vi "language.vi"(8 "Error In":errorcluster, 11 "QLocale In":refnum<class "QLocale.lvclass">) -> (0 "Error Out":errorcluster, 2 "Value":T1 items=["AnyLanguage", "C", "Abkhazian", "Oromo", "Afar", "Afrikaans", "Albanian", "Amharic", "Arabic", "Armenian", "Assamese", "Aymara", "Azerbaijani", "Bashkir", "Basque", "Bengali", "Dzongkha", "Bihari", "Bislama", "Breton", "Bulgarian", "Burmese", "Belarusian", "Khmer", "Catalan", "Chinese", "Corsican", "Croatian", "Czech", "Danish", "Dutch", "English", "Esperanto", "Estonian", "Faroese", "Fijian", "Finnish", "French", "WesternFrisian", "Gaelic", "Galician", "Georgian", "German", "Greek", "Greenlandic", "Guarani", "Gujarati", "Hausa", "Hebrew", "Hindi", "Hungarian", "Icelandic", "Indonesian", "Interlingua", "Interlingue", "Inuktitut", "Inupiak", "Irish", "Italian", "Japanese", "Javanese", "Kannada", "Kashmiri", "Kazakh", "Kinyarwanda", "Kirghiz", "Korean", "Kurdish", "Rundi", "Lao", "Latin", "Latvian", "Lingala", "Lithuanian", "Macedonian", "Malagasy", "Malay", "Malayalam", "Maltese", "Maori", "Marathi", "Marshallese", "Mongolian", "NauruLanguage", "Nepali", "NorwegianBokmal", "Occitan", "Oriya", "Pashto", "Persian", "Polish", "Portuguese", "Punjabi", "Quechua", "Romansh", "Romanian", "Russian", "Samoan", "Sango", "Sanskrit", "Serbian", "Ossetic", "SouthernSotho", "Tswana", "Shona", "Sindhi", "Sinhala", "Swati", "Slovak", "Slovenian", "Somali", "Spanish", "Sundanese", "Swahili", "Swedish", "Sardinian", "Tajik", "Tamil", "Tatar", "Telugu", "Thai", "Tibetan", "Tigrinya", "Tongan", "Tsonga", "Turkish", "Turkmen", "Tahitian", "Uighur", "Ukrainian", "Urdu", "Uzbek", "Vietnamese", "Volapuk", "Welsh", "Wolof", "Xhosa", "Yiddish", "Yoruba", "Zhuang", "Zulu", "NorwegianNynorsk", "Bosnian", "Divehi", "Manx", "Cornish", "Akan", "Konkani", "Ga", "Igbo", "Kamba", "Syriac", "Blin", "Geez", "Koro", "Sidamo", "Atsam", "Tigre", "Jju", "Friulian", "Venda", "Ewe", "Walamo", "Hawaiian", "Tyap", "Nyanja", "Filipino", "SwissGerman", "SichuanYi", "Kpelle", "LowGerman", "SouthNdebele", "NorthernSotho", "NorthernSami", "Taroko", "Gusii", "Taita", "Fulah", "Kikuyu", "Samburu", "Sena", "NorthNdebele", "Rombo", "Tachelhit", "Kabyle", "Nyankole", "Bena", "Vunjo", "Bambara", "Embu", "Cherokee", "Morisyen", "Makonde", "Langi", "Ganda", "Bemba", "Kabuverdianu", "Meru", "Kalenjin", "Nama", "Machame", "Colognian", "Masai", "Soga", "Luyia", "Asu", "Teso", "Saho", "KoyraChiini", "Rwa", "Luo", "Chiga", "CentralMoroccoTamazight", "KoyraboroSenni", "Shambala", "Bodo", "Avaric", "Chamorro", "Chechen", "Church", "Chuvash", "Cree", "Haitian", "Herero", "HiriMotu", "Kanuri", "Komi", "Kongo", "Kwanyama", "Limburgish", "LubaKatanga", "Luxembourgish", "Navaho", "Ndonga", "Ojibwa", "Pali", "Walloon", "Aghem", "Basaa", "Zarma", "Duala", "JolaFonyi", "Ewondo", "Bafia", "MakhuwaMeetto", "Mundang", "Kwasio", "Nuer", "Sakha", "Sangu", "CongoSwahili", "Tasawaq", "Vai", "Walser", "Yangben", "Avestan", "Asturian", "Ngomba", "Kako", "Meta", "Ngiemboon", "Aragonese", "Akkadian", "AncientEgyptian", "AncientGreek", "Aramaic", "Balinese", "Bamun", "BatakToba", "Buginese", "Buhid", "Carian", "Chakma", "ClassicalMandaic", "Coptic", "Dogri", "EasternCham", "EasternKayah", "Etruscan", "Gothic", "Hanunoo", "Ingush", "LargeFloweryMiao", "Lepcha", "Limbu", "Lisu", "Lu", "Lycian", "Lydian", "Mandingo", "Manipuri", "Meroitic", "NorthernThai", "OldIrish", "OldNorse", "OldPersian", "OldTurkish", "Pahlavi", "Parthian", "Phoenician", "PrakritLanguage", "Rejang", "Sabaean", "Samaritan", "Santali", "Saurashtra", "Sora", "Sylheti", "Tagbanwa", "TaiDam", "TaiNua", "Ugaritic", "Akoose", "Lakota", "StandardMoroccanTamazight", "Mapuche", "CentralKurdish", "LowerSorbian", "UpperSorbian", "Kenyang", "Mohawk", "Nko", "Prussian", "Kiche", "SouthernSami", "LuleSami", "InariSami", "SkoltSami", "Warlpiri", "ManichaeanMiddlePersian", "Mende", "AncientNorthArabian", "LinearA", "HmongNjua", "Ho", "Lezghian", "Bassa", "Mono", "TedimChin", "Maithili", "Ahom", "AmericanSignLanguage", "ArdhamagadhiPrakrit", "Bhojpuri", "HieroglyphicLuwian", "LiteraryChinese", "Mazanderani", "Mru", "Newari", "NorthernLuri", "Palauan", "Papiamento", "Saraiki", "TokelauLanguage", "TokPisin", "TuvaluLanguage", "UncodedLanguages", "Cantonese", "Osage", "Tangut"], 3 "QLocale Out":refnum<class "QLocale.lvclass">)   [LabVIEW 2014, in "QLocale.lvclass"]
doc: "LabVIEW-specific documentation is not yet available. See <b>https://doc.qt.io/qt-5/qlocale.html#language</b>"
uses:
  QLocale.lvclass
  Language.ctl
  LQSerialData/LQSerialData.lvclass/LQSerialData.ctl
  LQ Core.lvlib
  LQSerialData/LQSerialData.lvclass
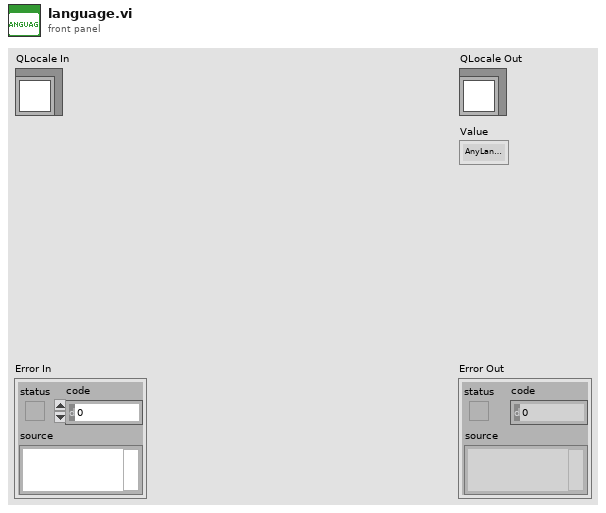
[diagram p1: front panel]
types:
  T1 = typedef "QLocale.lvclass/Language.ctl" = i32
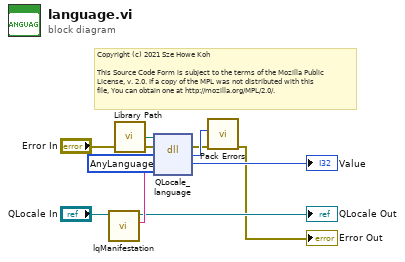
[diagram p0: block diagram]
diagram:
  w8 = T1 0 items=["AnyLanguage", "C", "Abkhazian", "Oromo", "Afar", "Afrikaans", "Albanian", "Amharic", "Arabic", "Armenian", "Assamese", "Aymara", "Azerbaijani", "Bashkir", "Basque", "Bengali", "Dzongkha", "Bihari", "Bislama", "Breton", "Bulgarian", "Burmese", "Belarusian", "Khmer", "Catalan", "Chinese", "Corsican", "Croatian", "Czech", "Danish", "Dutch", "English", "Esperanto", "Estonian", "Faroese", "Fijian", "Finnish", "French", "WesternFrisian", "Gaelic", "Galician", "Georgian", "German", "Greek", "Greenlandic", "Guarani", "Gujarati", "Hausa", "Hebrew", "Hindi", "Hungarian", "Icelandic", "Indonesian", "Interlingua", "Interlingue", "Inuktitut", "Inupiak", "Irish", "Italian", "Japanese", "Javanese", "Kannada", "Kashmiri", "Kazakh", "Kinyarwanda", "Kirghiz", "Korean", "Kurdish", "Rundi", "Lao", "Latin", "Latvian", "Lingala", "Lithuanian", "Macedonian", "Malagasy", "Malay", "Malayalam", "Maltese", "Maori", "Marathi", "Marshallese", "Mongolian", "NauruLanguage", "Nepali", "NorwegianBokmal", "Occitan", "Oriya", "Pashto", "Persian", "Polish", "Portuguese", "Punjabi", "Quechua", "Romansh", "Romanian", "Russian", "Samoan", "Sango", "Sanskrit", "Serbian", "Ossetic", "SouthernSotho", "Tswana", "Shona", "Sindhi", "Sinhala", "Swati", "Slovak", "Slovenian", "Somali", "Spanish", "Sundanese", "Swahili", "Swedish", "Sardinian", "Tajik", "Tamil", "Tatar", "Telugu", "Thai", "Tibetan", "Tigrinya", "Tongan", "Tsonga", "Turkish", "Turkmen", "Tahitian", "Uighur", "Ukrainian", "Urdu", "Uzbek", "Vietnamese", "Volapuk", "Welsh", "Wolof", "Xhosa", "Yiddish", "Yoruba", "Zhuang", "Zulu", "NorwegianNynorsk", "Bosnian", "Divehi", "Manx", "Cornish", "Akan", "Konkani", "Ga", "Igbo", "Kamba", "Syriac", "Blin", "Geez", "Koro", "Sidamo", "Atsam", "Tigre", "Jju", "Friulian", "Venda", "Ewe", "Walamo", "Hawaiian", "Tyap", "Nyanja", "Filipino", "SwissGerman", "SichuanYi", "Kpelle", "LowGerman", "SouthNdebele", "NorthernSotho", "NorthernSami", "Taroko", "Gusii", "Taita", "Fulah", "Kikuyu", "Samburu", "Sena", "NorthNdebele", "Rombo", "Tachelhit", "Kabyle", "Nyankole", "Bena", "Vunjo", "Bambara", "Embu", "Cherokee", "Morisyen", "Makonde", "Langi", "Ganda", "Bemba", "Kabuverdianu", "Meru", "Kalenjin", "Nama", "Machame", "Colognian", "Masai", "Soga", "Luyia", "Asu", "Teso", "Saho", "KoyraChiini", "Rwa", "Luo", "Chiga", "CentralMoroccoTamazight", "KoyraboroSenni", "Shambala", "Bodo", "Avaric", "Chamorro", "Chechen", "Church", "Chuvash", "Cree", "Haitian", "Herero", "HiriMotu", "Kanuri", "Komi", "Kongo", "Kwanyama", "Limburgish", "LubaKatanga", "Luxembourgish", "Navaho", "Ndonga", "Ojibwa", "Pali", "Walloon", "Aghem", "Basaa", "Zarma", "Duala", "JolaFonyi", "Ewondo", "Bafia", "MakhuwaMeetto", "Mundang", "Kwasio", "Nuer", "Sakha", "Sangu", "CongoSwahili", "Tasawaq", "Vai", "Walser", "Yangben", "Avestan", "Asturian", "Ngomba", "Kako", "Meta", "Ngiemboon", "Aragonese", "Akkadian", "AncientEgyptian", "AncientGreek", "Aramaic", "Balinese", "Bamun", "BatakToba", "Buginese", "Buhid", "Carian", "Chakma", "ClassicalMandaic", "Coptic", "Dogri", "EasternCham", "EasternKayah", "Etruscan", "Gothic", "Hanunoo", "Ingush", "LargeFloweryMiao", "Lepcha", "Limbu", "Lisu", "Lu", "Lycian", "Lydian", "Mandingo", "Manipuri", "Meroitic", "NorthernThai", "OldIrish", "OldNorse", "OldPersian", "OldTurkish", "Pahlavi", "Parthian", "Phoenician", "PrakritLanguage", "Rejang", "Sabaean", "Samaritan", "Santali", "Saurashtra", "Sora", "Sylheti", "Tagbanwa", "TaiDam", "TaiNua", "Ugaritic", "Akoose", "Lakota", "StandardMoroccanTamazight", "Mapuche", "CentralKurdish", "LowerSorbian", "UpperSorbian", "Kenyang", "Mohawk", "Nko", "Prussian", "Kiche", "SouthernSami", "LuleSami", "InariSami", "SkoltSami", "Warlpiri", "ManichaeanMiddlePersian", "Mende", "AncientNorthArabian", "LinearA", "HmongNjua", "Ho", "Lezghian", "Bassa", "Mono", "TedimChin", "Maithili", "Ahom", "AmericanSignLanguage", "ArdhamagadhiPrakrit", "Bhojpuri", "HieroglyphicLuwian", "LiteraryChinese", "Mazanderani", "Mru", "Newari", "NorthernLuri", "Palauan", "Papiamento", "Saraiki", "TokelauLanguage", "TokPisin", "TuvaluLanguage", "UncodedLanguages", "Cantonese", "Osage", "Tangut"] ("retVal")
  # "Copyright (c) 2021 Sze Howe Koh\n\nThis Source Code Form is subject to the terms of the Mozilla Public\nLicense, v. 2.0. If a copy of the MPL was not distributed with this\nfile, You can obtain one at http://mozilla.org/MPL/2.0/."
  n1 = call "lqManifestation.vi"("LQSerialData in"="QLocale In") -> ("Manifestation"=w7:string, "LQSerialData out"=→"QLocale Out":refnum<class "QLocale.lvclass">)  [unwired: 9 in]
  n2 = call "Library Path.vi"() -> ("Library Path"=w4:path)
  n3 = dll-call lib="?" fn="QLocale_language"(path in=w4, error in="Error In", "_retVal"=w8, "_instance"=w7) -> (error out=w2:errorcluster, w3:i32, "_retVal"=→"Value":i32)  [unwired: 2 in, 1 out]
  n4 = call "Pack Errors.vi"("Error In"=w2, "Error Code"=w3) -> ("Error Out"=→"Error Out":errorcluster)  [unwired: 9 in]
